vi "Get New Goal If Needed.vi"(8 "Current Goal":cluster{"X":dbl, "Y":dbl}, 11 "Obstacle Avoidance Data":T1={"LIDAR Data"={array[569 elements], array[569 elements]}, "dt"=0.0, "Wall Left?"=FALSE, "Encoder-Estimated Absolute Position"={"X"=0.0, "Y"=0.0}}) -> (0 "Next Goal":cluster{"X":dbl, "Y":dbl})   [LabVIEW 2017]
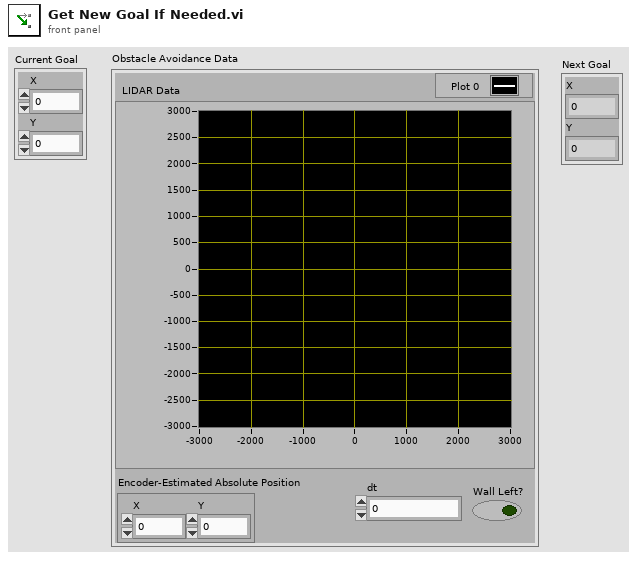
[diagram p1: front panel]
types:
  T1 = cluster{"LIDAR Data":cluster{dbl[], dbl[]}, "dt":dbl, "Wall Left?":bool, "Encoder-Estimated Absolute Position":cluster{"X":dbl, "Y":dbl}}
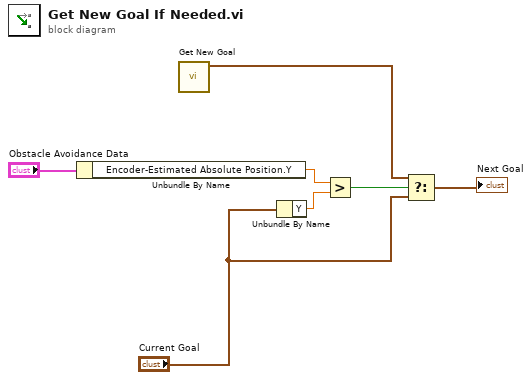
[diagram p0: block diagram]
diagram:
  n1 = Unbundle By Name("Obstacle Avoidance Data") -> ("Encoder-Estimated Absolute Position.Y"=w2:dbl)
  n2 = call "Get New Goal.vi"() -> ("New Goal"=w1:cluster{"X":dbl, "Y":dbl})  [unwired: 11 in]
  n3 = Unbundle By Name("Current Goal") -> ("Y"=w5:dbl)
  n4 = Greater?(x=w2, y=w5) -> (0:w4:bool)
  n5 = Select(t=w1, s=w4, f="Current Goal") -> (s? t:f=→"Next Goal":cluster{"X":dbl, "Y":dbl})
